vi "FSM_Delete.vi"(8 "error in (no error)":errorcluster, 11 "FSM":refnum<class "FSM.lvclass">) -> (0 "error out":errorcluster)   [LabVIEW 2021, in "FSM.lvclass"]
doc: "Author: J. Camilo Gomez C."
uses:
  FSM.lvclass
  FSM.lvclass/FSM.ctl
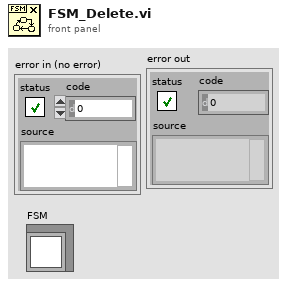
[diagram p1: front panel]
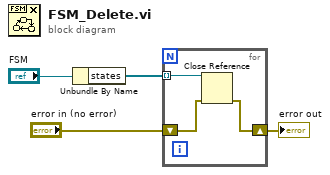
[diagram p0: block diagram]
diagram:
  n1 = Unbundle By Name("FSM") -> ("states"=w3:refnum<vi>[])
  n2 = for {
    tunnel: w3 -> [w7] mode=indexing
    shift-right: [w5] -> w1
    shift-left: "error in (no error)" -> [w6]
    n3 = Close Reference(reference=w7, error in (no error)=w6) -> (error out=w5:errorcluster)
  }
  "error out" <- w1
